vi "Get Best Fit Output v2.vi"(8 "error in":errorcluster, 9 "Optimal Offset Selection Criterion":T1, 11 "Array of Fit Outputs":T2[](array[typedef])) -> (0 "Error Out":errorcluster, 1 "optimal index":i32, 3 "Best Fit Output":T2={"best nonlinear fit"=[], "best fit parameters"=[], "R^2"=0.0, "RMSE"=0.0, "error out"={"status"=FALSE, "code"=0, "source"=""}, "Fitting Method"=enum."Least Square", "number of function calls"=0, "number of iterations"=0, "covariance"=[], "Chi 2"=0.0, "DOF"=0, "Fit Convergence Criterion"=enum."Continue", "Fitting Algorithm"=enum."Levenberg-Marquardt", "Weighted Fit"=enum."Unweighted", "Gradient"=0.0, "|Delta Chi 2|"=0.0, "|Delta Chi 2|/Chi 2"=0.0, "Max |Delta a| /|a|"=0.0, "Lambda"=-1.0, "RSS"=0.0, "AIC"=0.0, "BIC"=0.0, "Max number of function calls"=0, "Max number of iterations"=0, "IRF"={"X Array"=[], "Y Array"=[]}, "IRF Normalization Factor"=0.0, "Decay Normalization Factor"=0.0, "Number of offset fits"=0, "Weighted Chi2"=-1.0, "Unweighted Chi2"=-1.0})   [LabVIEW 2021, in "Fits.lvlib"]
doc: "Picks the fit with the largest R^2"
uses:
  Fits.lvlib
  Non-linear Fit Output v4.ctl
  Nonlinear Fit Method.ctl
  <vilib>/Analysis/Matrix/Datatypes/RealMatrix.ctl
  Convergence Criteria.ctl
  Non-linear Fitting Algorithm.ctl
  IRF(X)PSED/Fit Weights Type v2.ctl
  Graphs/XY Graph/XY Graph Plot Data.ctl
  Optimal Offset Selection Criterion.ctl
  <vilib>/Analysis/Matrix/NI_Matrix.lvlib
  Graphs/XY Graph/XY Graph Add-Ons.lvlib
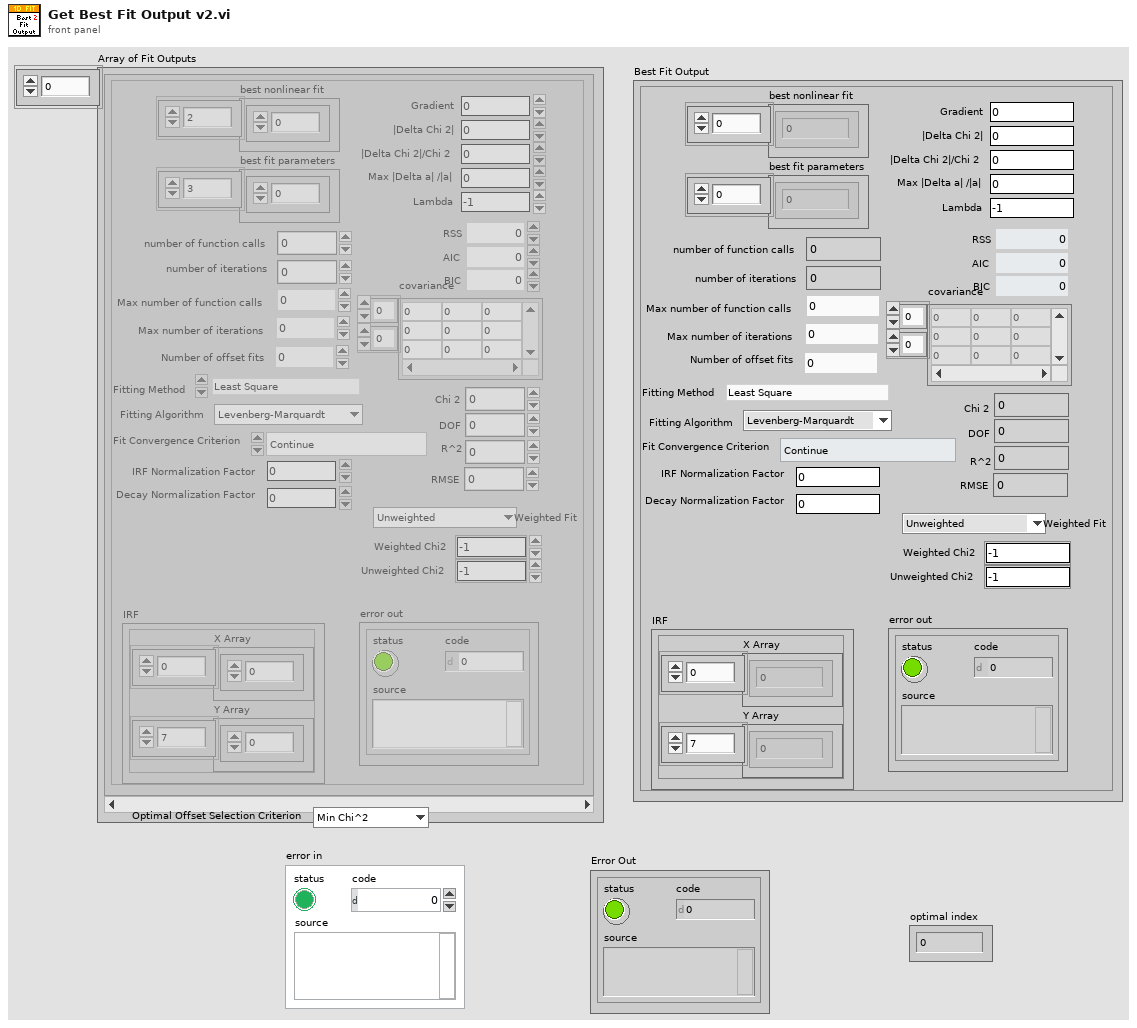
[diagram p1: front panel]
types:
  T1 = typedef "Fits.lvlib/Optimal Offset Selection Criterion.ctl" = enum16{"Min Chi^2", "Max R^2"}
  T2 = typedef "Fits.lvlib/Non-linear Fit Output v4.ctl" = cluster{"best nonlinear fit":dbl[], "best fit parameters":dbl[], "R^2":dbl, "RMSE":dbl, "error out":errorcluster, "Fitting Method":T3, "number of function calls":i32, "number of iterations":i32, "covariance":T4, "Chi 2":dbl, "DOF":i32, "Fit Convergence Criterion":T5, "Fitting Algorithm":T6, "Weighted Fit":T7, "Gradient":dbl, "|Delta Chi 2|":dbl, "|Delta Chi 2|/Chi 2":dbl, "Max |Delta a| /|a|":dbl, "Lambda":dbl, "RSS":dbl, "AIC":dbl, "BIC":dbl, "Max number of function calls":i32, "Max number of iterations":i32, "IRF":T8, "IRF Normalization Factor":dbl, "Decay Normalization Factor":dbl, "Number of offset fits":i32, "Weighted Chi2":dbl, "Unweighted Chi2":dbl}
  T3 = typedef "Fits.lvlib/Nonlinear Fit Method.ctl" = enum16{"Least Square", "Least Absolute Residual", "Bisquare", "MLE"}
  T4 = typedef "NI_Matrix.lvlib/RealMatrix.ctl" = dbl[][]
  T5 = typedef "Fits.lvlib/Convergence Criteria.ctl" = enum16{"Continue", "Tolerances Exceeded", "Max Time Exceeded", "Max Iterations Exceeded", "Max Function Evaluations Exceeded", "Scale Range Exceeded"}
  T6 = typedef "Fits.lvlib/Non-linear Fitting Algorithm.ctl" = enum16{"Levenberg-Marquardt", "Trust-Region Dogleg"}
  T7 = typedef "Fits.lvlib/Fit Weights Type v2.ctl" = enum16{"Unweighted", "1/Variance (Neyman)", "1/Variance (Pearson)", "Best of All"}
  T8 = typedef "XY Graph Add-Ons.lvlib/XY Graph Plot Data.ctl" = cluster{"X Array":dbl[], "Y Array":dbl[]}
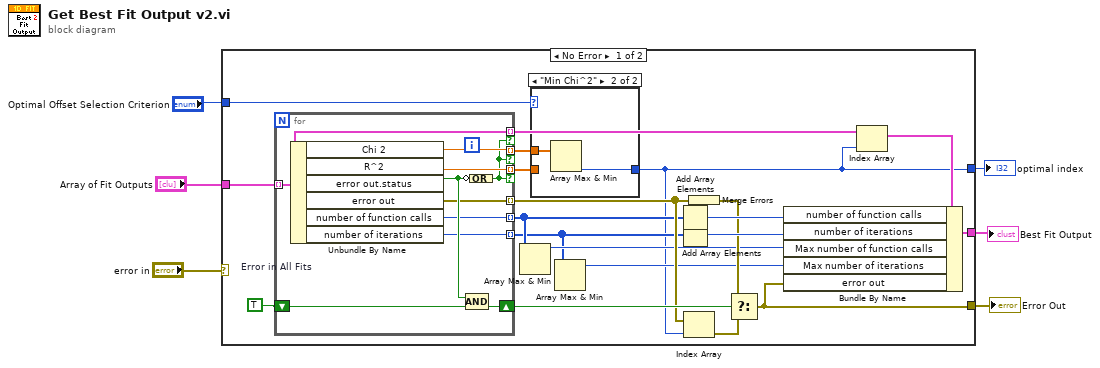
[diagram p0: block diagram]
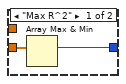
[diagram p2: hidden frame]
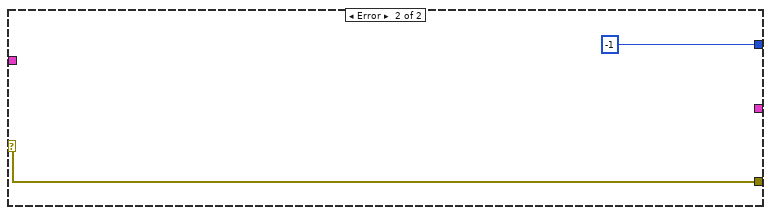
[diagram p3: hidden frame]
diagram:
  n1 = case shown="No Error" "error in" {
    selector: "error in" -> [_ w42]
    tunnel: [w22 _] -> w6
    tunnel: "Array of Fit Outputs" -> [w14 _]
    tunnel: [w17 w42] -> w5
    tunnel: [w9 -1] -> w4
    tunnel: "Optimal Offset Selection Criterion" -> [w8 _]
    frame No Error {
      w26 = TRUE  # Error in All Fits
      n2 = for {
        tunnel: w14 -> [w33] mode=indexing
        tunnel: [w40] -> w21 mode=indexing if=w31
        shift-right: [w38] -> w19
        shift-left: w26 -> [w37]
        tunnel: [w36] -> w16 mode=indexing
        tunnel: [w33] -> w25 mode=indexing if=w31
        tunnel: [w35] -> w13 mode=indexing
        tunnel: [w34] -> w11 mode=indexing
        tunnel: [w32] -> w7 mode=indexing if=w31
        n3 = Unbundle By Name(w33) -> ("Chi 2"=w32:dbl, "R^2"=w40:dbl, "error out.status"=w39:bool, "error out"=w36:errorcluster, "number of function calls"=w35:i32, "number of iterations"=w34:i32)
        n4 = Compound Arithmetic op=AND(w39, w37) -> (w38:bool)
        n5 = Compound Arithmetic op=OR(invert w39) -> (w31:bool)
      }
      n6 = Array Max & Min(array=w13) -> (max value=w12:i32)  [unwired: 3 out]
      n7 = case shown="\"Min Chi^2\"" w8 {
        tunnel: w21 -> [w28 _]
        tunnel: [w27 w29] -> w9
        tunnel: w7 -> [_ w30]
        frame "Max R^2" {
          n8 = Array Max & Min(array=w28) -> (max index (indices)=w27:i32)  [unwired: 3 out]
        }
        frame "Min Chi^2" {
          n9 = Array Max & Min(array=w30) -> (min index (indices)=w29:i32)  [unwired: 3 out]
        }
      }
      n10 = Array Max & Min(array=w11) -> (max value=w10:i32)  [unwired: 3 out]
      n11 = Add Array Elements(numeric array=w13) -> (sum=w24:i32)
      n12 = Add Array Elements(numeric array=w11) -> (sum=w23:i32)
      n13 = Index Array(array=w16, index=w9) -> (element=w15:errorcluster)
      n14 = Merge Errors(w16) -> (w18:errorcluster)
      n15 = Select(t=w18, s=w19, f=w15) -> (s? t:f=w17:errorcluster)
      n16 = Index Array(array=w25, index=w9) -> (element=w20:T2)
      n17 = Bundle By Name(cluster=w20, "number of function calls"=w24, "number of iterations"=w23, "Max number of function calls"=w12, "Max number of iterations"=w10, "error out"=w17) -> (w22:T2)
    }
    frame Error {
    }
  }
  "Best Fit Output" <- w6
  "Error Out" <- w5
  "optimal index" <- w4
